vi "fgv_NtripClient_errors.vi"(7 "cmd":enum16{"init", "read", "write"}(ring), 8 "error in":errorcluster, 11 "Error led":T1={"GNSS Serial"=0, "NMEA val"=0, "Send Serial"=0, "Ntrip TCP"=0, "RTCM val"=0, "GMAP"=0, "TBD1"=2, "TBD2"=2, "TBD3"=2}) -> (0 "error out":errorcluster, 3 "Error led out":T1={"GNSS Serial"=0, "NMEA val"=0, "Send Serial"=0, "Ntrip TCP"=0, "RTCM val"=0, "GMAP"=0, "TBD1"=2, "TBD2"=2, "TBD3"=2})   [LabVIEW 2019]
uses:
  Ctrl/Ntrip error-leds.ctl
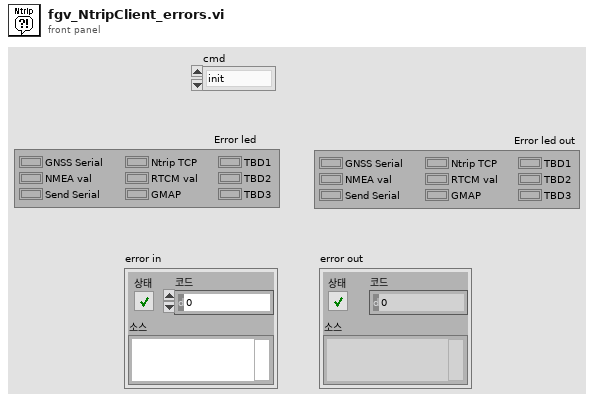
[diagram p1: front panel]
types:
  T1 = typedef "Ntrip error-leds.ctl" = cluster{"GNSS Serial":u8, "NMEA val":u8, "Send Serial":u8, "Ntrip TCP":u8, "RTCM val":u8, "GMAP":u8, "TBD1":u8, "TBD2":u8, "TBD3":u8}
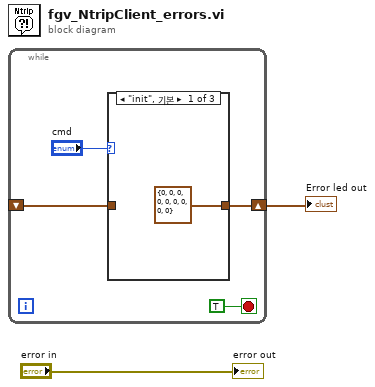
[diagram p0: block diagram]
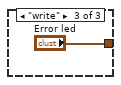
[diagram p3: hidden frame]
diagram:
  n1 = while {
    shift-right: [w4] -> w1
    shift-left: _ -> [w3]
    stop <- TRUE stop-if-true
    n2 = case shown="\"init\", 기본" "cmd" {
      tunnel: [T1 {"GNSS Serial"=0, "NMEA val"=0, "Send Serial"=0, "Ntrip TCP"=0, "RTCM val"=0, "GMAP"=0, "TBD1"=0, "TBD2"=0, "TBD3"=0} ("Error led") w8 "Error led"] -> w4
      tunnel: w3 -> [_ w8 _]
      frame "init", Default {
      }
      frame "read" {
      }
      frame "write" {
      }
    }
  }
  "Error led out" <- w1
  "error out" <- "error in"
